vi "GetSimInfo.vi"(6 "Slot":T1, 8 "error in (no error)":errorcluster caption="错误输入（无错误）", 9 "MEID":string, 10 "Data":string[][](array[string])=[["8986031490021881534", "460036161669975", "2A645416CB435F94", "8006A127", "460036161669975@mycdma.cn", "DB60264368A1D188", "18101891253", "A1000021A59070"], ["8986031490021881535", "460036161669976", "32FA5764D69C76BE", "80FAE4E6", "460036161669976@mycdma.cn", "B3AA1B3D2F0D5593", "18964872399", "A1000021A58D61"], ["", "", "", "", "", "", "", ""], ["", "", "", "", "", "", "", ""], ["", "", "", "", "", "", "", ""], ["", "", "", "", "", "", "", ""], ["", "", "", "", "", "", "", ""], ["", "", "", "", "", "", "", ""], ["", "", "", "", "", "", "", ""], ["", "", "", "", "", "", "", ""], ["", "各位，模块烧号主要是写五码，包括IMSI、AKEY、MEID（ESN）、AN(EVDO USER)、AAA(EVDO PWD)。", "", "", "", "", "", ""], ["", "其中ESN和MEID在模块出厂时已经写入，两者均可通过AT指令读取，但ESN不可更改。", "", "", "", "", "", ""], ["", "经询问及实际测试，上海电信绑定ESN号而广东电信未绑定，意味着上海电信五码烧录到其它模块是不可用的，但广东电信则无此限制。", "", "", "", "", "", ""], ["", "", "", "", "", "", "", ""], ["", "", "", "", "", "", "", ""], ["", "目前已确定跟上海电信合作，后续模块及卡号使用过程中，如遇到模块损坏，则意味着该卡必须销号（除非向电信申请绑定新的ESN），否则烧录到其它模块中是没用的。", "", "", "", "", "", ""]]) -> (0 "error out":errorcluster caption="错误输出", 2 "SIMInfo":T2, 3 "Result":bool)   [LabVIEW 2013]
uses:
  SystemCode/SysControl/Slot.ctl
  GlobalValue.vi
panel:
  out "SIM信息":string[](array[string])
  in  "已删除的部分":string[](array[string])=["ICCID", "IMSI", "AKEY", "ESN", "EVDO账号", "EVDO密码", "MDN", "MEID"]
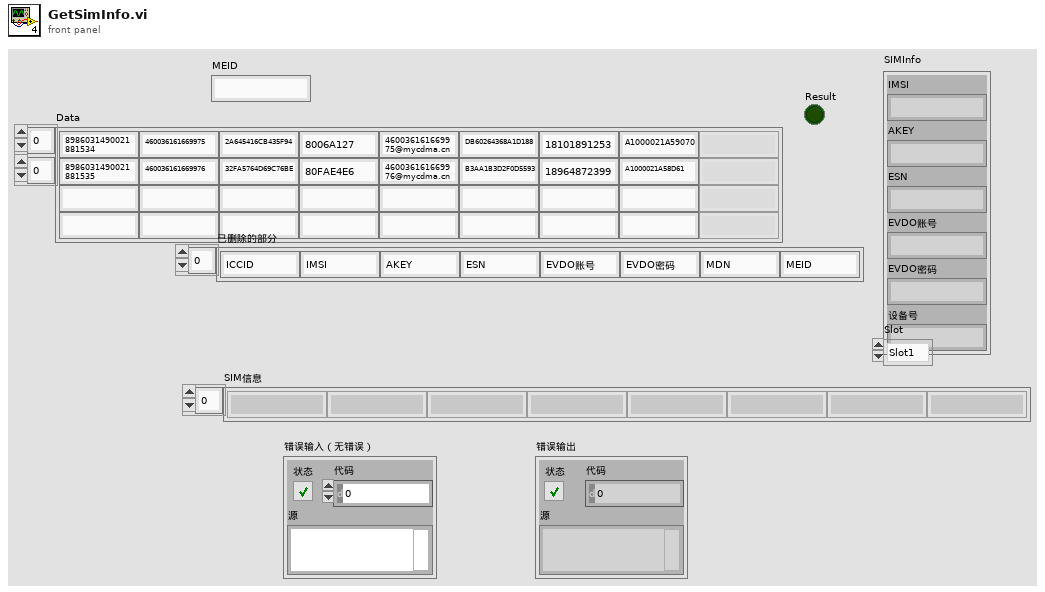
[diagram p1: front panel]
types:
  T1 = typedef "Slot.ctl" = enum16{"Slot1", "Slot2", "Slot3", "Slot4"}
  T2 = cluster{"IMSI":string, "AKEY":string, "ESN":string, "EVDO账号":string, "EVDO密码":string, "设备号":string}
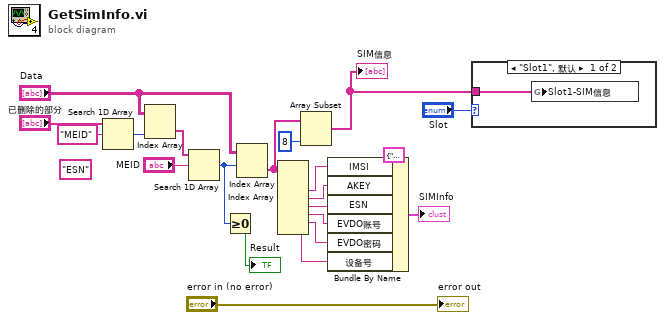
[diagram p0: block diagram]
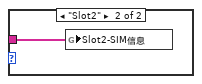
[diagram p2: hidden frame]
diagram:
  (unwired) "ESN" ("元素")
  n1 = Search 1D Array(1D array="已删除的部分", element="MEID" ("元素")) -> (index of element=w19:i32)  [unwired: 1 in]
  n2 = Index Array(array="Data", index (col)=w19) -> (element=w18:string[])  [unwired: 1 in]
  n3 = Search 1D Array(1D array=w18, element="MEID") -> (index of element=w2:i32)  [unwired: 1 in]
  n4 = Greater Or Equal To 0?(x=w2) -> (x >= 0?=→"Result":bool)
  n5 = Index Array(array="Data", index (row)=w2) -> (element=w5:string[])  [unwired: 1 in]
  n6 = Index Array(array=w5) -> (element #2=w15:string, element #3=w14:string, element #4=w13:string, element #5=w12:string, element #6=w11:string, element #7=w8:string)  [unwired: 7 in, 1 out]
  n7 = Array Subset(array=w5, length=8 ("长度")) -> (w4:string[])  [unwired: 1 in]
  "SIM信息" <- w4
  n8 = Bundle By Name(cluster=T2 {"IMSI"="460036161699998", "AKEY"="F20DF5B495104E47", "ESN"="808A93DA", "EVDO账号"="460036161699998@mycdma.cn ", "EVDO密码"="3E5A5E78927F5458", "设备号"="3E5A5E78927F5458"} ("SIMInfo"), "IMSI"=w15, "AKEY"=w14, "ESN"=w13, "EVDO账号"=w12, "EVDO密码"=w11, "设备号"=w8) -> (→"SIMInfo":T2)
  n9 = case shown="\"Slot1\", 默认" "Slot" {
    tunnel: w4 -> [w22 w23]
    frame "Slot1", Default {
      n10 = global write "GlobalValue.vi" "Slot1-SIM信息"(w22) -> ()
    }
    frame "Slot2" {
      n11 = global write "GlobalValue.vi" "Slot2-SIM信息"(w23) -> ()
    }
  }
  "error out" <- "error in (no error)"
